vi "Graph GetYScale.vi"(8 "err in":errorcluster, 11 "GraphChart入力":refnum<vi>) -> (0 "err out":errorcluster, 2 "Y軸データ":T1(array[cluster]), 3 "Y軸名称":string[](array[string]))   [LabVIEW 2014]
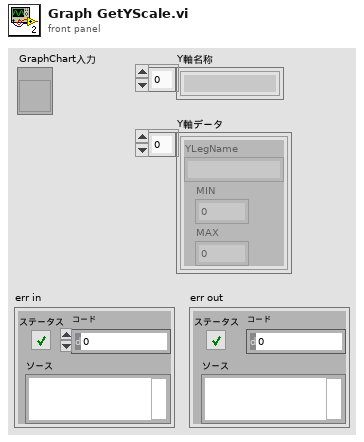
[diagram p1: front panel]
types:
  T1 = cluster{"YLegName":string, "MIN":dbl, "MAX":dbl}[]
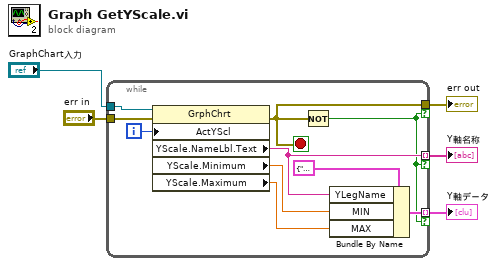
[diagram p0: block diagram]
diagram:
  n1 = while {
    tunnel: "GraphChart入力" -> [w15]
    tunnel: [w11] -> w3 mode=indexing if=w7
    tunnel: [w13] -> w2 if=w7
    tunnel: [w8] -> w4 mode=indexing if=w7
    tunnel: "err in" -> [w6]
    i -> [w14]
    stop <- w13 stop-if-true
    n2 = property class="GrphChrt"(reference=w15, error in=w6, "ActYScl"=w14) -> (error out=w13:errorcluster, "YScale.NameLbl.Text"=w11:string, "YScale.Minimum"=w10:dbl, "YScale.Maximum"=w9:dbl)  [unwired: 1 out]
    n3 = Not(x=w13) -> (.not. x?=w7:bool)
    n4 = Bundle By Name(cluster=cluster{"YLegName":string, "MIN":dbl, "MAX":dbl} {"YLegName"="", "MIN"=0.0, "MAX"=0.0} ("クラスタ"), "YLegName"=w11, "MIN"=w10, "MAX"=w9) -> (w8:cluster{"YLegName":string, "MIN":dbl, "MAX":dbl})
  }
  "Y軸データ" <- w4
  "Y軸名称" <- w3
  "err out" <- w2
